vi "play-AFM-CS-imaging.vi"() -> ()   [LabVIEW 2017]
uses:
  z-axis-params.ctl
  controls/boolean_info.ctl
  <userlib>/_matio/level5/Public/MAT-File Data Types.ctl
  <vilib>/userdefined/High Color/nirio_resource_hc.ctl
  controls/expMetaData.ctl
  <vilib>/Utility/file.llb/Read Delimited Spreadsheet (DBL).vi
  <vilib>/FPGAPlugInAG/cRIO-9082/niLvFpga_Open_cRIO-9082.vi
  <vilib>/rvi/interface/common/dynamic/niFpgaDynamicAddResources.vi
  <vilib>/FPGAPlugInAG/Dynamic/niLvFpga_Reset_Dynamic.vi
  <vilib>/rvi/interface/common/niFpgaWaitOnOcc.vi
  <vilib>/Utility/error.llb/Error Cluster From Error Code.vi
  <vilib>/rvi/errors/niLvFpgaAdjustHostInterfaceError.vi
  <vilib>/FPGAPlugInAG/Dynamic/niLvFpga_Run_Dynamic.vi
  <vilib>/Utility/file.llb/Write Delimited Spreadsheet (DBL).vi
  <vilib>/FPGAPlugInAG/Dynamic/niLvFpga_Close_Dynamic.vi
  <userlib>/_matio/level5/Public/Write/Append Data Element.llb/Append Data Element (Anything).vi
  <vilib>/rvi/interface/nirviOpenFPGA/nirviOpenFPGA.xnode
  FPGA Bitfiles/afmimagingcontro_FPGATargetSPARTA_cs-scanningaltzt_AOdy1tOC72s.lvbitx
  <vilib>/rvi/interface/nirviMethod/nirviMethod.xnode
  <vilib>/rvi/interface/nirviReadWriteControl/nirviReadWriteControl.xnode
  <vilib>/rvi/interface/nirviCloseFPGA/nirviCloseFPGA.xnode
  <vilib>/FPGAPlugInAG/Dynamic/niLvFpga_ConfigureFifo_Dynamic.vi
  <vilib>/rvi/errors/niLvFpgaMergeErrorWithErrorCode.vi
  <vilib>/rvi/interface/Simulation/niFpgaSimulationCallBeginRW.vi
  <vilib>/FPGAPlugInAG/Dynamic/niLvFpga_ReadFifo_Dynamic.vi
  NiFpgaLv.dll
  <userlib>/_matio/level5.lvlib
  <vilib>/FPGAPlugInAG/Dynamic/niLvFpga_WriteFifo_Dynamic.vi
panel:
  out "input-data-path":path
  in  "Kiz_down":sgl=0.001
  in  "max_Z_settle_samples":i16=5000
  out "boolean \nindicators":T1
  in  "Den":sgl[](array[numeric])=[1.0, -1.0, 0.0, 0.0, 0.0, 0.0, 0.0, 0.0, 0.0]
  in  "Num":sgl[](array[numeric])=[0.01, 0.0, 0.0, 0.0, 0.0, 0.0, 0.0, 0.0, 0.0]
  out "CS Time":dbl
  out "Current Case":i16
  out "state times":dbl[](array[numeric])
  out "iter":i32
  out "entity-index":i16
  out "x = 0?":bool
  out "Numeric":i32
  out "error out 2":errorcluster
  in  "Tab Control":T2(tab)
  in  "init Z up":sgl step=0.5
  in  "trigger-0":bool
  in  "numEntities":i16
  in  "data-root":path=path "C:/Users/arnold/Documents/labview/afm_imaging/data/cs-data"
  in  "z-axis-params":T3={"TOL"=0.3, "ramp_rate"=-5e-05, "z_u_max"=5.0, "setpoint"=0.0, "Ki"=0.01, "Z_error_threshold"=0.05, "Z_settled_samples_threshold "=500, "z_UP"=1.5, "zup_N"=500, "TF Order"=1, "Num"=[1.0, 0.0, 0.0, 0.0, 0.0, 0.0, 0.0, 0.0, 0.0], "Den"=[1.0, 0.0, 0.0, 0.0, 0.0, 0.0, 0.0, 0.0, 0.0]} {"Z_error_threshold" format="%#_13g"; "ramp_rate" format="%#_4g"; "TOL" format="%#_13g"}
  in  "step_down_frac":fxp<+,8,1>=1.0
  in  "input-file-name":string="cs-traj-5perc-500nm-5mic-1Hz.csv"
  out "output-data-path":path
  out "output-meta-data-path":path
  in  "note-blob":string
  in  "overwrite":bool
  in  "TsTicks":u32=1600
  in  "Ki-xy":sgl=0.005
  in  "collect all":bool
  in  "collect move":bool
  in  "do_Alt_Ztrigger":bool
  in  "do_xy_CL":bool
  in  "xy settled-samples\n threshold":i16=200
  in  "xy error-threshold":sgl=0.1
  out "number-settled-samples-x":i16
  out "number-settled-samples-y":i16
  out "case-selected":i16
  out "number-settled-samples-Z":i16
  out "size(s)":i32
  out "nsamps":i32
  out "elements left":i32=1
  out "y iter":i32
  out "size(s) 2":i32[](array[numeric])
  out "Array":i32[][](array[numeric])
  out "z-control":dbl[](graph)
  out "x-axis":dbl[](graph)
  out "z-error":dbl[](graph)
  out "y-axis":dbl[](graph)
  in  "STOP":bool
  # "- If collect all = fasle and collect move = false,\nwe only collect measurement data.\n- If collect all = false, and collect move = true,\nwe collect measurement and move data.\n- If collect all = true, we collect everything."
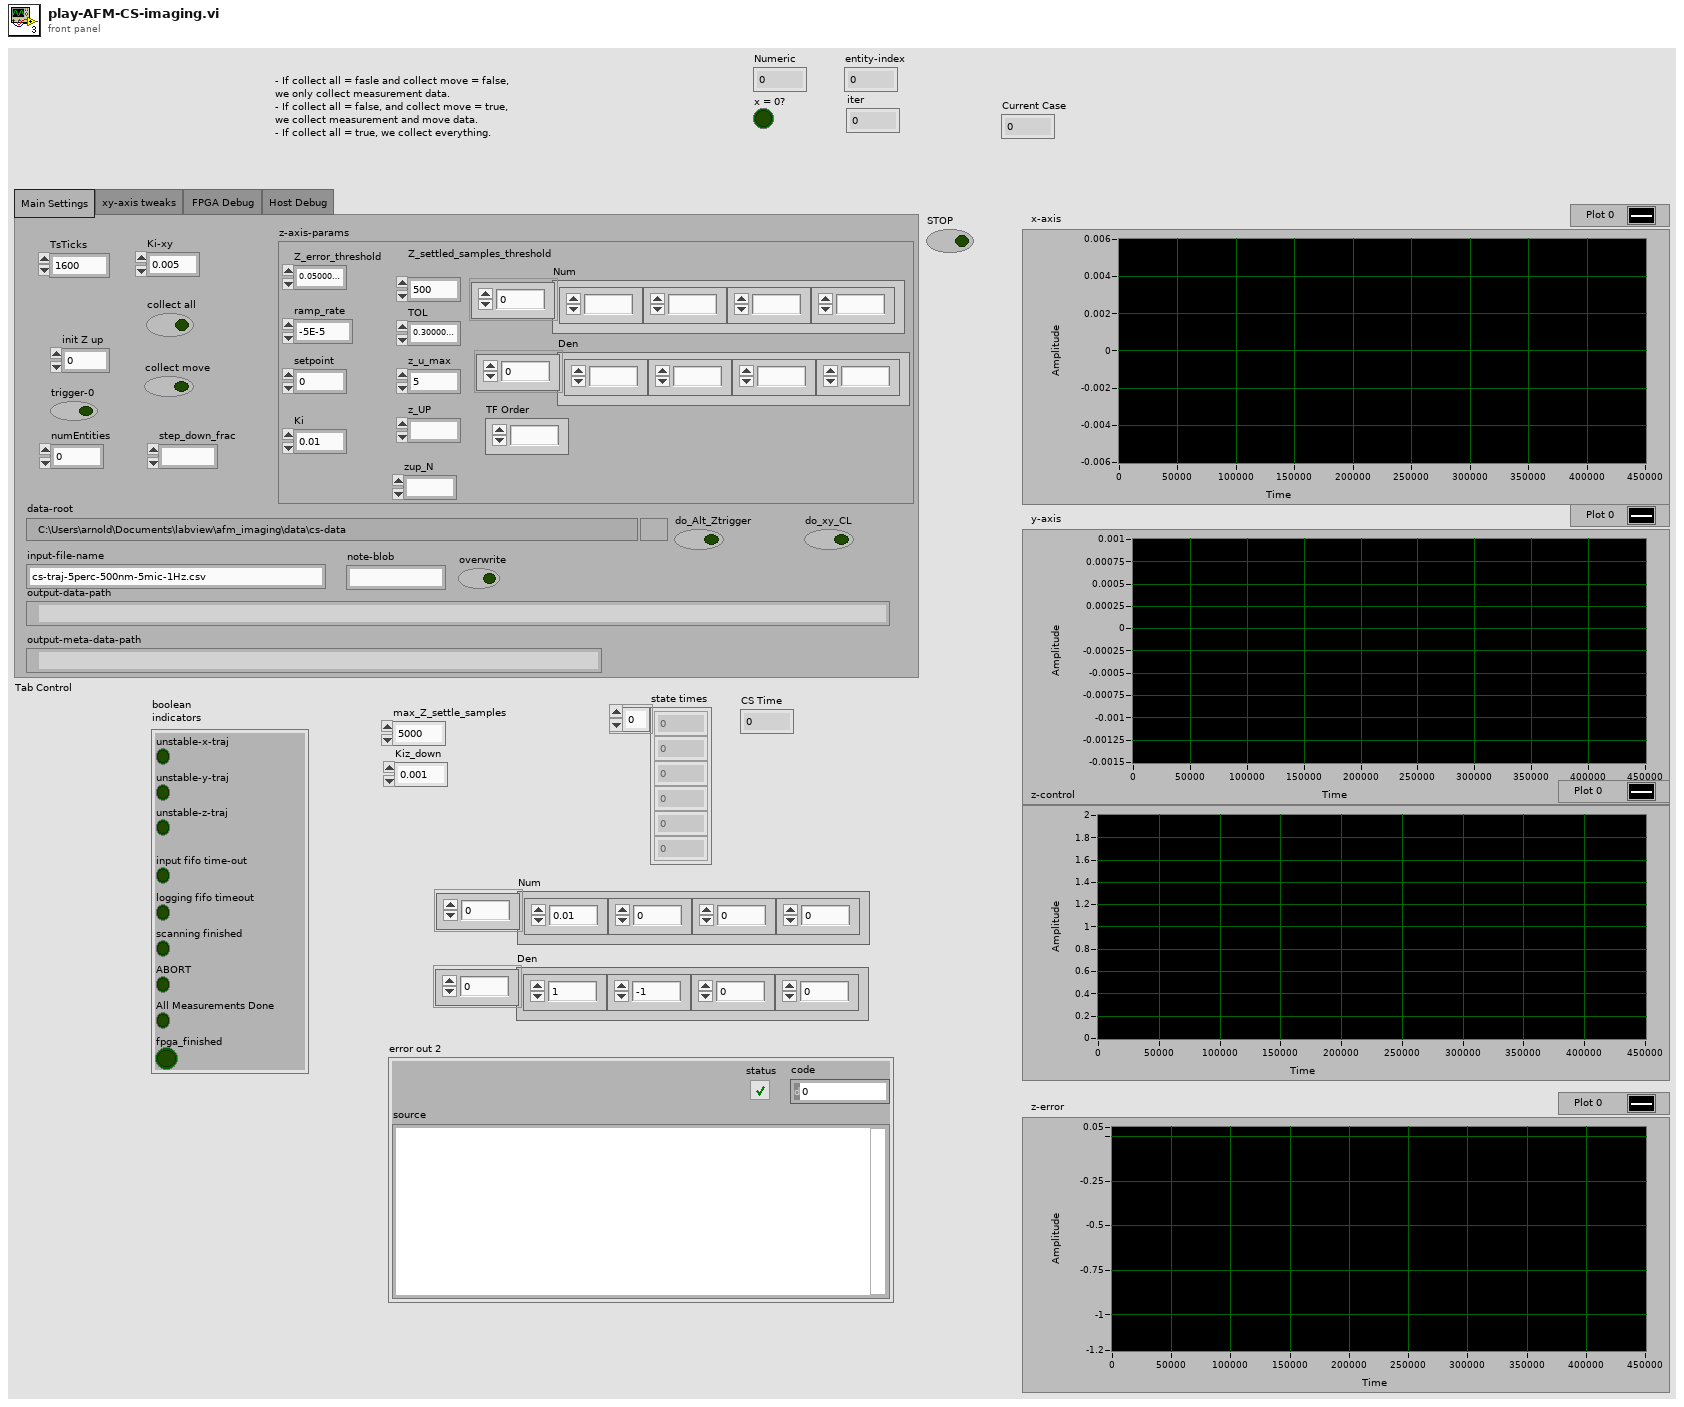
[diagram p1: front panel]
types:
  T1 = typedef "boolean_info.ctl" = cluster{"unstable-z-traj":bool, "input fifo time-out":bool, "logging fifo timeout":bool, "scanning finished":bool, "unstable-x-traj":bool, "unstable-y-traj":bool, "ABORT":bool, "All Measurements Done":bool, "fpga_finished":bool}
  T2 = enum32{"Main Settings", "xy-axis tweaks", "FPGA Debug ", "Host Debug"}
  T3 = typedef "z-axis-params.ctl" = cluster{"TOL":sgl, "ramp_rate":sgl, "z_u_max":sgl, "setpoint":sgl, "Ki":sgl, "Z_error_threshold":sgl, "Z_settled_samples_threshold ":i16, "z_UP":fxp<+/-,16,5>, "zup_N":i16, "TF Order":i32, "Num":sgl[], "Den":sgl[]}
  T4 = typedef "level5.lvlib/MAT-File Data Types.ctl" = enum32{"_invalid", "miINT8", "miUINT8", "miINT16", "miUINT16", "miINT32", "miUINT32", "miSINGLE", "_reserved_1", "miDOUBLE", "_reserved_2", "_reserved_3", "miINT64", "miUINT64", "miMATRIX", "miCOMPRESSED", "miUTF8", "miUTF16", "miUTF32"}
  T5 = typedef "nirio_resource_hc.ctl" = tag
  T6 = cluster{"unstable-z-traj":bool, "input fifo time-out":bool, "logging fifo timeout":bool, "scanning finished":bool, "unstable-x-traj":bool, "unstable-y-traj":bool, "ABORT":bool, "All Measurements Done":bool, "fpga_finished":bool}
  T7 = enum16{"open", "replace", "create", "open or create", "replace or create", "replace or create with confirmation"}
  T8 = typedef "expMetaData.ctl" = cluster{"xy_error_threshold":sgl, "xy_settled_samples_threshold":i16, "Ki_xy":sgl, "state_counts":dbl[], "TOL":sgl, "ramp_rate":sgl, "z_u_max":sgl, "setpoint":sgl, "Ki":sgl, "Z_error_threshold":sgl, "Z_settled_samples_threshold ":i16, "z_UP":sgl, "zup_N":i16, "Num":sgl[], "Den":sgl[], "max_Z_settle_samples":i16, "Kiz_down":sgl, "do_xy_CL":bool, "do_Alt_Ztrigger":bool, "output-data-path":path, "input-data-path":path}
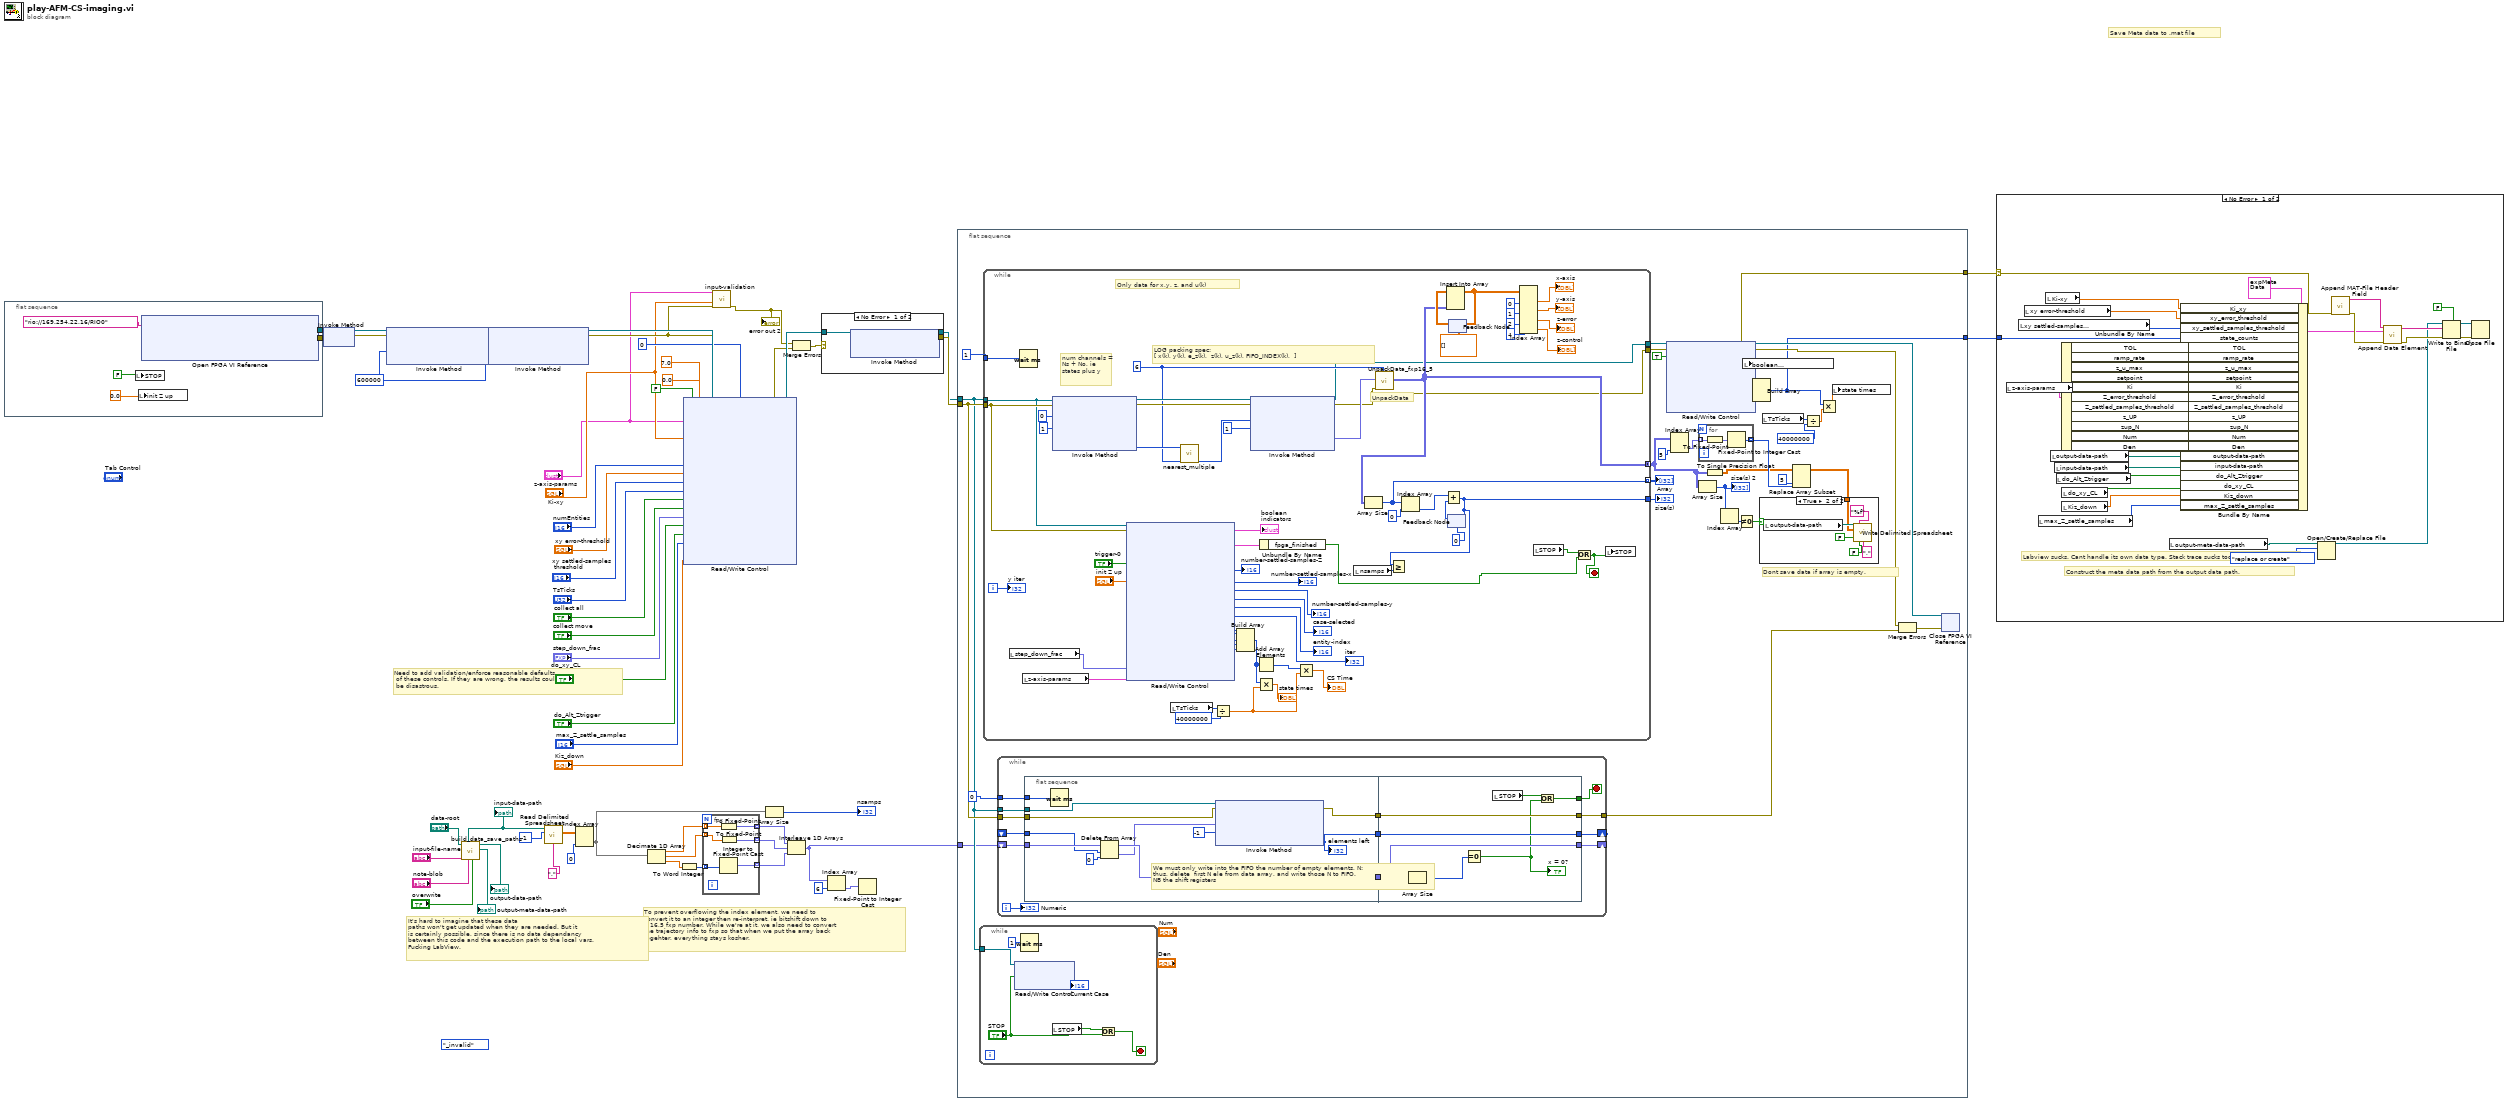
[diagram p0: block diagram]
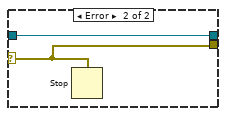
[diagram p4: hidden frame]
diagram:
  (unwired) MAT-File_Data_Types."_invalid" ("MAT-File Data Types")
  w56 = 600000
  # "It's hard to imagine that these data\npaths won't get updated when they are needed. But it \nis certainly possible, since there is no data dependancy \nbetween this code and the execution path to the local vars.\nFucking LabView."
  # "Save Meta data to .mat file"
  # "To prevent overflowing the index element, we need to \nconvert it to an integer then re-interpret, ie bitshift down to \na 16,5 fxp number. While we're at it, we also need to convert\nthe trajectory info to fxp so that when we put the array back\ntogehter, everything stays kosher."
  # "Need to add validation/enforce reasonable defaults\n of these controls. If they are wrong, the results could\n be disastrous."
  n1 = flat-sequence {
    tunnel: [w62] -> w55
    tunnel: [w61] -> w54
    frame #0 {
      n2 = local write "STOP"(FALSE) -> ()
      n3 = local write "init Z up"(0.0) -> ()
      n4 = xnode "Open FPGA VI Reference"("resource name"=T5 "rio://169.254.22.16/RIO0") -> ("FPGA VI Reference Out"=w62:refnum<k20>, "error out"=w61:errorcluster)  [unwired: 1 in]
    }
  }
  n5 = xnode "Invoke Method"("FPGA VI Reference In"=w55, "error in"=w54) -> ("FPGA VI Reference Out"=w48:refnum<k20>, "error out"=w47:errorcluster)
  n6 = xnode "Invoke Method"("FPGA VI Reference In"=w48, "error in"=w47, "Requested Depth"=w56) -> ("FPGA VI Reference Out"=w50:refnum<k20>, "error out"=w51:errorcluster)  [unwired: 1 out]
  n7 = call "build_data_save_paths.vi"("overwrite"="overwrite", "note-blob"="note-blob", "base-file-name"="input-file-name", "data-root"="data-root") -> ("output-meta-data-path"=→"output-meta-data-path":path, "output-data-path"=→"output-data-path":path, "input-data-path"=w7:path)  [unwired: 3 in, 2 out]
  "input-data-path" <- w7
  n8 = xnode "Invoke Method"("FPGA VI Reference In"=w50, "error in"=w51, "Requested Depth"=w56) -> ("FPGA VI Reference Out"=w57:refnum<k20>, "error out"=w33:errorcluster)  [unwired: 1 out]
  n9 = call-poly <vilib>:"Read Delimited Spreadsheet.vi"("file path (dialog if empty)"=w7, "number of rows (all:-1)"=-1, "delimiter (\\t)"=",") -> ("all rows"=w42:dbl[][])  [unwired: 7 in, 5 out]
  n10 = Index Array(array=w42, index (col)=0 ("dimension size")) -> (element=w18:dbl[])  [unwired: 1 in]
  n11 = Decimate 1D Array(w18) -> (w26:dbl[], w25:dbl[], w27:dbl[])
  n12 = To Word Integer(number=w27) -> (16bit integer=w24:i16[])
  n13 = xnode "Read/Write Control"("FPGA VI Reference In"=w57, "error in"=w33, "initial case"=i16 0, "z-axis-params"="z-axis-params", "xy-bound"=sgl 7.0, "Ki-xy"="Ki-xy", "init Z up"=sgl 0.0 ("u(0)"), "trigger-0"=FALSE, "numEntities"="numEntities", "xy-error-threshold"="xy error-threshold", "settled-samples threshold"="xy settled-samples\n threshold", "TsTicks"="TsTicks", "collect all"="collect all", "collect move"="collect move", "step_down_frac"="step_down_frac", "do_xy_CL"="do_xy_CL", "do_orig_Ztrigger"="do_Alt_Ztrigger", "max_Z_settle_samples"="max_Z_settle_samples", "Kiz_down"="Kiz_down") -> ("FPGA VI Reference Out"=w49:refnum<k20>, "error out"=w30:errorcluster)  [unwired: 1 out]
  n14 = for {
    tunnel: w26 -> [w68] mode=indexing
    tunnel: w25 -> [w67] mode=indexing
    tunnel: [w66] -> w22 mode=indexing
    tunnel: [w65] -> w23 mode=indexing
    tunnel: w24 -> [w64] mode=indexing
    tunnel: [w63] -> w21 mode=indexing
    n15 = Integer to Fixed-Point Cast(integer=w64) -> (fixed-point=w63:fxp<+/-,16,5>)  [unwired: 1 in]
    n16 = To Fixed-Point(number=w68) -> (fixed-point=w65:fxp<+/-,16,5>)  [unwired: 1 in]
    n17 = To Fixed-Point(number=w67) -> (fixed-point=w66:fxp<+/-,16,5>)  [unwired: 1 in]
  }
  n18 = call "input-validation.vi"("error constant"=w33, "Ki-xy"="Ki-xy", "z-axis-params"="z-axis-params") -> ("error out"=w29:errorcluster)  [unwired: 8 in]
  "error out 2" <- w29
  n19 = Array Size(array=w18) -> (size(s)=→"nsamps":i32)
  n20 = Interleave 1D Arrays(w23, w22, w21) -> (w17:fxp<+/-,16,5>[])
  n21 = Merge Errors(w29, w30) -> (w28:errorcluster)
  n22 = case shown="No Error" w28 {
    selector: w28 -> [_ w72]
    tunnel: [w71 w72] -> w52
    tunnel: w49 -> [w70 w73]
    tunnel: [w69 w73] -> w40
    frame No Error {
      n23 = xnode "Invoke Method"("FPGA VI Reference In"=w70) -> ("FPGA VI Reference Out"=w69:refnum<k20>, "error out"=w71:errorcluster)  [unwired: 2 in]
    }
    frame Error {
      n24 = Stop(stop? (T)=w72) -> ()
    }
  }
  n25 = Index Array(array=w17, index=6) -> (element=w20:fxp<+/-,16,5>)
  n26 = Fixed-Point to Integer Cast(1:w20) -> ()  [unwired: 1 out]
  n27 = flat-sequence {
    tunnel: w52 -> [w104]
    tunnel: w40 -> [w98]
    tunnel: w17 -> [w96]
    tunnel: [w84] -> w14
    tunnel: [w74] -> w13
    frame #0 {
      # "Dont save data if array is empty."
      n28 = while {
        tunnel: w98 -> [w123]
        stop <- w119 stop-if-true
        n29 = xnode "Read/Write Control"("FPGA VI Reference In"=w123, "ABORT"="STOP") -> ("Current Case"=→"Current Case":i16)  [unwired: 1 in, 2 out]
        n30 = Wait (ms)(milliseconds to wait=u32 1) -> ()  [unwired: 1 out]
        n31 = local read "STOP"() -> (w120:bool)
        n32 = Or(x=w120, y="STOP") -> (x .or. y?=w119:bool)
      }
      n33 = while {
        tunnel: 1 -> [w214]
        tunnel: w98 -> [w202]
        tunnel: w104 -> [w203]
        tunnel: [w167] -> w102
        tunnel: [w178] -> w91 mode=concatenating
        tunnel: [w200] -> w107
        tunnel: [w176] -> w101
        tunnel: [w193] -> w97 mode=indexing
        i -> [w201]
        stop <- w194 stop-if-true
        w179 = u32 6 ("y")
        # "LOG packing spec:\n[ x(k), y(k), e_z(k),  z(k), u_z(k), FIFO_INDEX(k),  ]"
        # "num channels = Ns + No, ie states plus y"
        # "Only data for x,y, z, and u(k)"
        # "UnpackData"
        n34 = local read "step_down_frac"() -> (w155:fxp<+,8,1>)
        n35 = Wait (ms)(milliseconds to wait=w214) -> ()  [unwired: 1 out]
        n36 = local read "z-axis-params"() -> (w156:T3)
        n37 = xnode "Invoke Method"("FPGA VI Reference In"=w202, "error in"=w203, "Number of Elements"=0 ("Timeout (ms)"), "Timeout (ms)"=1) -> ("FPGA VI Reference Out"=w210:refnum<k20>, "error out"=w211:errorcluster, "Elements Remaining"=w197:u32)  [unwired: 1 out]
        n38 = xnode "Read/Write Control"("FPGA VI Reference In"=w202, "error in"=w203, "trigger-0"="trigger-0", "init Z up"="init Z up", "step_down_frac"=w155, "z-axis-params"=w156) -> ("boolean  indicators"=w160:T6, "number-settled-samples-Z"=→"number-settled-samples-Z":i16, "number-settled-samples-x"=→"number-settled-samples-x":i16, "number-settled-samples-y"=→"number-settled-samples-y":i16, "Current Case"=→"case-selected":i16, "entity-index"=→"entity-index":i16, "iter"=→"iter":i32, "state1-count"=w172:u64, "state2-count"=w171:u64, "state3-count"=w170:u64, "state4-count"=w169:u64, "state5-count"=w168:u64)  [unwired: 1 in, 2 out]
        "boolean \nindicators" <- w160
        n39 = local read "TsTicks"() -> (w163:u32)
        n40 = call "nearest_multiple.vi"("numChan"=w179, "N"=w197) -> ("(int) y*floor(x/y)"=w196:u64)  [unwired: 9 in]
        n41 = Divide(x=w163, y=u32 40000000) -> (x/y=w158:dbl)
        n42 = Build Array(w172, w171, w170, w169, w168) -> (w159:u64[])
        n43 = xnode "Invoke Method"("FPGA VI Reference In"=w210, "error in"=w211, "Number of Elements"=w196, "Timeout (ms)"=1) -> ("FPGA VI Reference Out"=w167:refnum<k20>, "error out"=w176:errorcluster, "Data"=w177:fxp<+/-,16,5>[])  [unwired: 1 out]
        n44 = Add Array Elements(numeric array=w159) -> (sum=w164:u64)
        n45 = Multiply(x=w159, y=w158) -> (x*y=→"state times":dbl[])
        n46 = Unbundle By Name(w160) -> ("fpga_finished"=w175:bool)
        n47 = Multiply(x=w164, y=w158) -> (x*y=→"CS Time":dbl)
        n48 = local read "nsamps"() -> (w207:i32)
        n49 = call "UnpackData_fxp16_5.vi"("NumChannels"=w179, "error In"=w176, "1D Data In"=w177) -> ("2D Data Out"=w178:fxp<+/-,16,5>[][])  [unwired: 7 in, 1 out]
        n50 = Array Size(array=w178) -> (size(s)=w193:i32[])
        n51 = Index Array(array=w193, index=0) -> (element=w205:i32)
        n52 = feedback #1(0) -> (w206:i32)
        n53 = Add(x=w205, y=w206) -> (x+y=w200:i32)
        n54 = Greater Or Equal?(x=w200, y=w207) -> ()  [unwired: 1 out]
        n55 = feedback-in #1(w200) -> ()
        n56 = feedback #2(dbl[][] []) -> (w189:dbl[][])
        n57 = Insert Into Array(array=w189, new element=w178) -> (w180:dbl[][])  [unwired: 2 in]
        n58 = feedback-in #2(w180) -> ()
        n59 = Index Array(array=w180, index (col) #1=0 ("disabled index (col)"), index (col) #2=1 ("index (col)"), index (col) #3=2 ("index (col)"), index (col) #4=4 ("index (col)")) -> (element #1=→"x-axis":dbl[], element #2=→"y-axis":dbl[], element #3=→"z-error":dbl[], element #4=→"z-control":dbl[])  [unwired: 4 in]
        n60 = local read "STOP"() -> (w195:bool)
        n61 = Or(x=w195, y=w175) -> (x .or. y?=w194:bool)
        n62 = local write "STOP"(w194) -> ()
        "y iter" <- w201
      }
      "size(s)" <- w107
      "Array" <- w97
      n63 = while {
        tunnel: [w134] -> w103
        tunnel: 0 -> [w136]
        shift-right: [w130] -> _
        shift-left: _ -> [w133]
        shift-right: [w128] -> _
        shift-left: w96 -> [w135]
        tunnel: w98 -> [w127]
        tunnel: w104 -> [w126]
        i -> [w124]
        stop <- w125 stop-if-true
        n64 = flat-sequence {
          tunnel: w136 -> [w147]
          tunnel: w135 -> [w142]
          tunnel: w133 -> [w138]
          tunnel: [w145] -> w132
          tunnel: [w143] -> w131
          tunnel: [w144] -> w129
          tunnel: w127 -> [w140]
          tunnel: w126 -> [w139]
          tunnel: [w154] -> w130
          tunnel: [w151] -> w134
          tunnel: w132 -> [w151]
          tunnel: w131 -> [w154]
          tunnel: w129 -> [w152]
          tunnel: [w152] -> w128
          tunnel: [w148] -> w125
          frame #0 {
            # "We must only write into the FIFO the number of empty elements, N:\nthus, delete  first N ele from data array, and write those N to FIFO.\nNB the shift registers"
            n65 = Wait (ms)(milliseconds to wait=w147) -> ()  [unwired: 1 out]
            n66 = Delete From Array(array=w142, length=w138, index=0) -> (deleted portion=w141:fxp<+/-,16,5>[], array with subset deleted=w144:fxp<+/-,16,5>[])
            n67 = xnode "Invoke Method"("FPGA VI Reference In"=w140, "error in"=w139, "Data"=w141, "Timeout (ms)"=-1) -> ("error out"=w145:errorcluster, "Empty Elements Remaining"=w143:u32)  [unwired: 1 out]
            "elements left" <- w143
          }
          frame #1 {
            n68 = Array Size(array=w152) -> (size(s)=w153:i32)
            n69 = Equal To 0?(x=w153) -> (x = 0?=w150:bool)
            "x = 0?" <- w150
            n70 = local read "STOP"() -> (w149:bool)
            n71 = Or(x=w149, y=w150) -> (x .or. y?=w148:bool)
          }
        }
        "Numeric" <- w124
      }
      n72 = xnode "Read/Write Control"("FPGA VI Reference In"=w102, "error in"=w101, "ABORT"=TRUE) -> ("FPGA VI Reference Out"=w99:refnum<k20>, "error out"=w84:errorcluster, "boolean  indicators"=w79:T6, "state1-count"=w89:u64, "state2-count"=w88:u64, "state3-count"=w87:u64, "state4-count"=w86:u64, "state5-count"=w85:u64)
      n73 = Index Array(array=w91, index (col)=5) -> (element=w94:fxp<+/-,16,5>[])  [unwired: 1 in]
      n74 = for {
        tunnel: w94 -> [w116] mode=indexing
        tunnel: [w117] -> w92 mode=indexing
        n75 = To Fixed-Point(number=w116) -> (fixed-point=w115:fxp<+/-,16,5>)  [unwired: 1 in]
        n76 = Fixed-Point to Integer Cast(1:w115) -> (0:w117:i16)
      }
      n77 = Array Size(array=w91) -> (size(s)=w80:i32[])
      "size(s) 2" <- w80
      n78 = To Single Precision Float(number=w91) -> (single precision float=w90:sgl[][])
      n79 = Index Array(array=w80) -> (element=w81:i32)  [unwired: 1 in]
      n80 = Not Equal To 0?(x=w81) -> (x != 0?=w82:bool)
      n81 = local write "boolean \nindicators"(w79) -> ()
      n82 = Build Array(w89, w88, w87, w86, w85) -> (w74:u64[])
      n83 = local read "TsTicks"() -> (w78:u32)
      n84 = Replace Array Subset(array=w90, new element=w92, index (col)=5) -> (w83:sgl[][])  [unwired: 1 in]
      n85 = case shown="True" w82 {
        tunnel: w83 -> [_ w109]
        frame False {
        }
        frame True {
          n86 = local read "output-data-path"() -> (w114:path)
          n87 = call-poly <vilib>:"Write Delimited Spreadsheet.vi"("file path (dialog if empty)"=w114, "format (%.3f)"="%f", "2D data"=w109, "append to file? (new file:F)"=FALSE, "transpose? (no:F)"=FALSE, "delimiter (\\t)"=",") -> ()  [unwired: 8 in, 2 out]
        }
      }
      n88 = Divide(x=w78, y=u32 40000000) -> (x/y=w76:dbl)
      n89 = Multiply(x=w74, y=w76) -> (x*y=w75:dbl[])
      n90 = local write "state times"(w75) -> ()
      n91 = Merge Errors(w84, w103) -> (w105:errorcluster)
      n92 = xnode "Close FPGA VI Reference"("FPGA VI Reference In"=w99, "error in"=w105) -> ()  [unwired: 1 out]
    }
  }
  n93 = case shown="No Error" w14 {
    selector: w14 -> [w242 _]
    tunnel: w13 -> [w229 _]
    frame No Error {
      # "Construct the meta data path from the output data path."
      # "Labview sucks. Cant handle its own data type. Stack trace sucks too."
      n94 = local read "z-axis-params"() -> (w228:T3)
      n95 = local read "xy settled-samples\n threshold"() -> (w225:i16)
      n96 = local read "xy error-threshold"() -> (w226:sgl)
      n97 = local read "max_Z_settle_samples"() -> (w216:i16)
      n98 = local read "Ki-xy"() -> (w227:sgl)
      n99 = local read "output-data-path"() -> (w220:path)
      n100 = local read "input-data-path"() -> (w219:path)
      n101 = local read "do_Alt_Ztrigger"() -> (w218:bool)
      n102 = Unbundle By Name(w228) -> ("TOL"=w239:sgl, "ramp_rate"=w238:sgl, "z_u_max"=w237:sgl, "setpoint"=w236:sgl, "Ki"=w235:sgl, "Z_error_threshold"=w234:sgl, "Z_settled_samples_threshold"=w233:i16, "z_UP"=w232:fxp<+/-,16,5>, "zup_N"=w231:i16, "Num"=w222:sgl[], "Den"=w221:sgl[])
      n103 = local read "do_xy_CL"() -> (w217:bool)
      n104 = local read "Kiz_down"() -> (w215:sgl)
      n105 = local read "output-meta-data-path"() -> (w223:path)
      n106 = Bundle By Name(cluster=T8 {"xy_error_threshold"=0.1, "xy_settled_samples_threshold"=200, "Ki_xy"=0.005, "state_counts"=[], "TOL"=0.3, "ramp_rate"=-5e-06, "z_u_max"=5.0, "setpoint"=0.0, "Ki"=0.001, "Z_error_threshold"=0.0, "Z_settled_samples_threshold "=0, "z_UP"=1.5, "zup_N"=5000, "Num"=[-0.00254, 0.000408, 0.00295, 0.0, 0.0, 0.0, 0.0, 0.0, 0.0], "Den"=[0.982758, -1.98194, 1.0, 0.0, 0.0, 0.0, 0.0, 0.0, 0.0], "max_Z_settle_samples"=5000, "Kiz_down"=0.001, "do_xy_CL"=FALSE, "do_Alt_Ztrigger"=FALSE, "output-data-path"=path "", "input-data-path"=path ""} ("ExpMetaData"), "Ki_xy"=w227, "xy_error_threshold"=w226, "xy_settled_samples_threshold"=w225, "state_counts"=w229, "TOL"=w239, "ramp_rate"=w238, "z_u_max"=w237, "setpoint"=w236, "Ki"=w235, "Z_error_threshold"=w234, "Z_settled_samples_threshold"=w233, "z_UP"=w232, "zup_N"=w231, "Num"=w222, "Den"=w221, "output-data-path"=w220, "input-data-path"=w219, "do_Alt_Ztrigger"=w218, "do_xy_CL"=w217, "Kiz_down"=w215, "max_Z_settle_samples"=w216) -> (w240:T8)
      n107 = Open/Create/Replace File(file path (use dialog)=w223, operation (0:open)=T7."replace or create") -> (refnum out=w241:refnum<file>)  [unwired: 4 in, 2 out]
      n108 = call <userlib>:"Append MAT-File Header Field.vi"("error"=w242) -> ("result string"=w249:string, "error out"=w243:errorcluster)  [unwired: 13 in]
      n109 = call-poly <userlib>:"Append Data Element.vi"("initial string"=w249, "data"=w240, "error in (no error)"=w243) -> ("result string"=w247:string, "error out"=w248:errorcluster)  [unwired: 11 in]
      n110 = Write to Binary File(file (use dialog)=w241, data=w247, error in=w248, 5:FALSE ("prepend array or string size? (T)")) -> (refnum out=w244:refnum<file>, error out=w245:errorcluster)  [unwired: 2 in, 1 out]
      n111 = Close File(refnum=w244, error in=w245) -> ()  [unwired: 2 out]
    }
    frame Error {
    }
  }
